vi "LEDS.vi"(7 "Action":T1, 8 "error in":errorcluster, 10 "On/Off":bool) -> (0 "error out":errorcluster)   [LabVIEW 2015]
uses:
  LEDSaction.ctl
  <vilib>/Rock Robotics/SystemInterfaces/DIO/FPGA_DIOChannel.ctl
  <vilib>/Rock Robotics/SystemInterfaces/Typedef/FPGA_TypedefDigitalModule.ctl
panel:
  out "PressureHigh":bool
  out "PressureLow":bool
  out "Shoot":bool
  out "Shift":bool
  out "Hot":bool
  out "NotHot":bool
  out "10 Seconds":bool
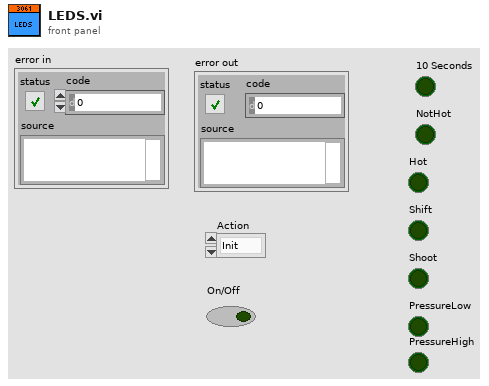
[diagram p1: front panel]
types:
  T1 = typedef "LEDSaction.ctl" = enum16{"Init", "10SecondsLeft", "LimitDown", "LimitUp", "CollectDown", "CollectUp", "NotHot", "Hot", "Shift", "RollBack", "RollFwd", "Shoot", "Distance Low", "DistanceHigh", "PressureLow", "PressureHigh"}
  T2 = typedef "FPGA_DIOChannel.ctl" = enum8{"DIO 1", "DIO 2", "DIO 3", "DIO 4", "DIO 5", "DIO 6", "DIO 7", "DIO 8", "DIO 9", "DIO 10", "DIO 11", "DIO 12", "DIO 13", "DIO 14", "Invalid"}
  T3 = typedef "FPGA_TypedefDigitalModule.ctl" = enum16{"Digital Module 1", "Digital Module 2"}
  T4 = typedef "WPI_DigitalOutputDevRef.ctl" = cluster{"Digital Module":T3, "DIO Channel":T2, "DevStatus":errorcluster}
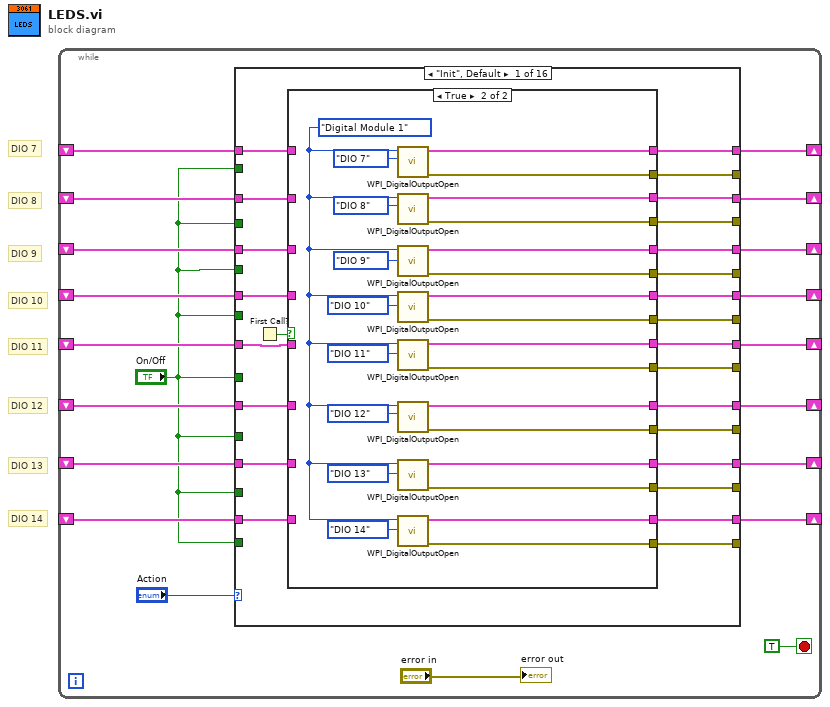
[diagram p0: block diagram]
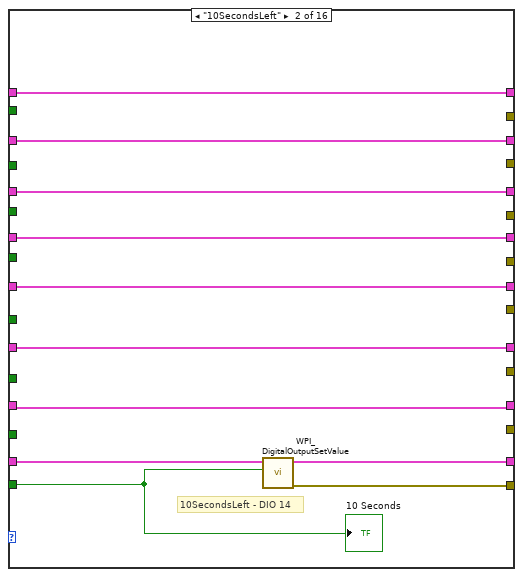
[diagram p3: hidden frame]
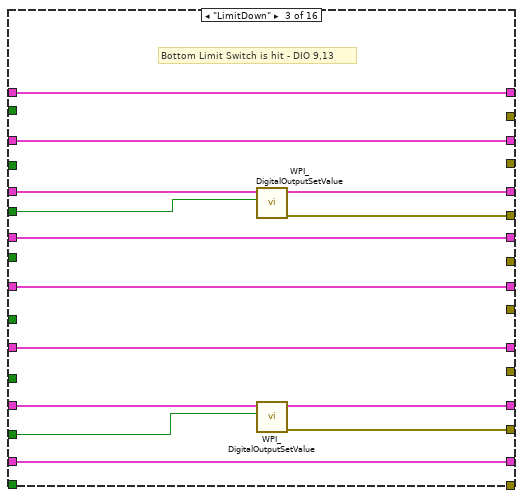
[diagram p4: hidden frame]
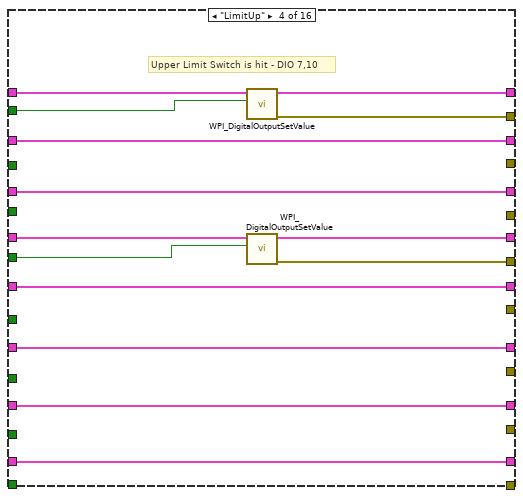
[diagram p5: hidden frame]
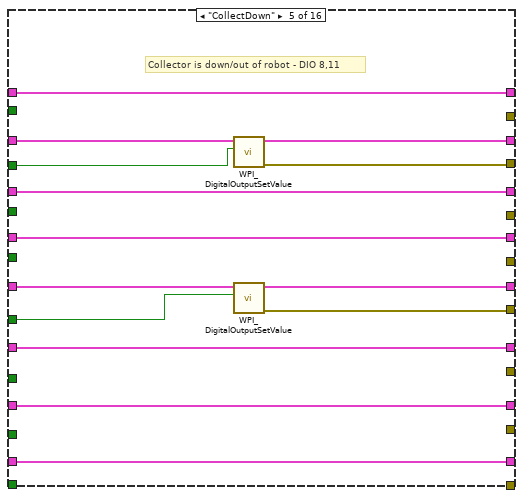
[diagram p6: hidden frame]
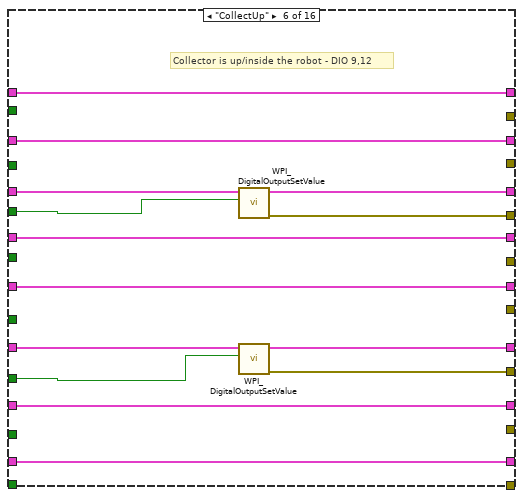
[diagram p7: hidden frame]
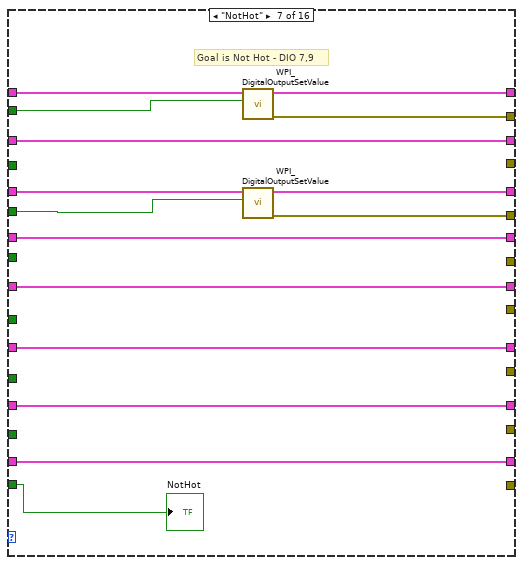
[diagram p8: hidden frame]
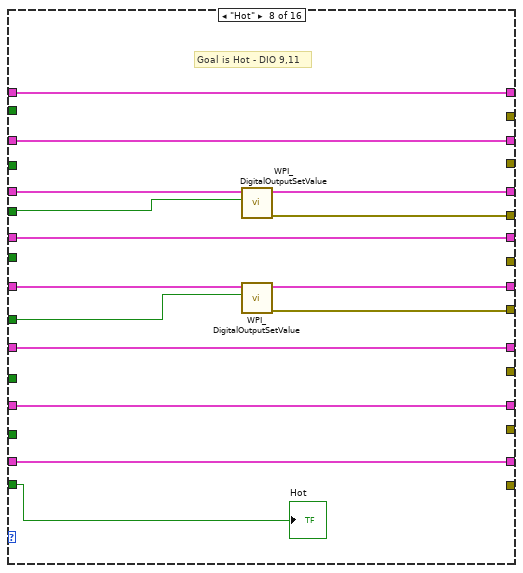
[diagram p9: hidden frame]
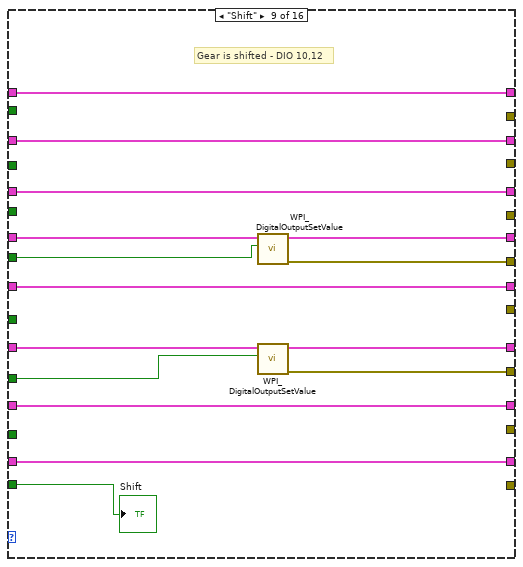
[diagram p10: hidden frame]
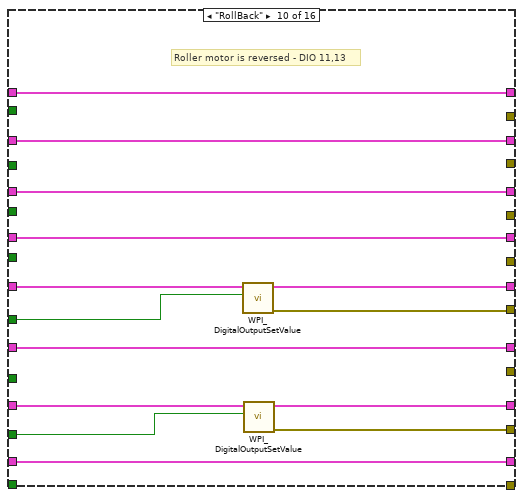
[diagram p11: hidden frame]
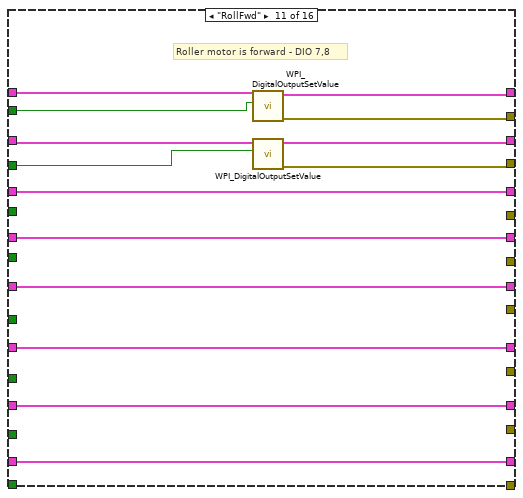
[diagram p12: hidden frame]
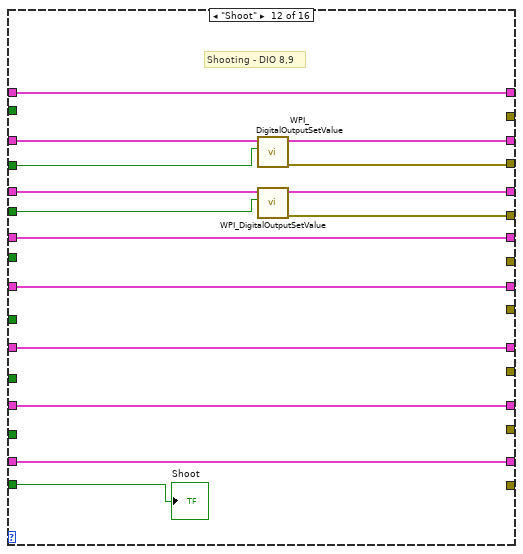
[diagram p13: hidden frame]
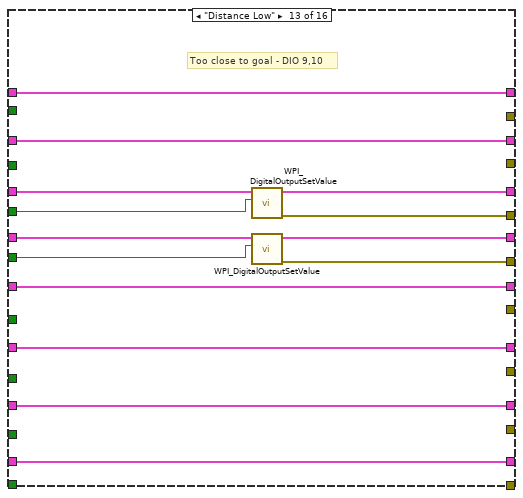
[diagram p14: hidden frame]
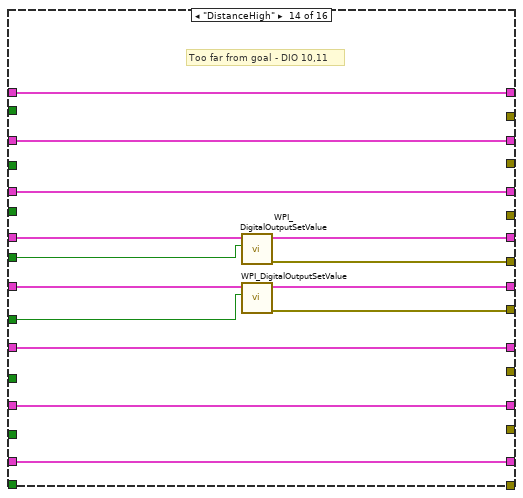
[diagram p15: hidden frame]
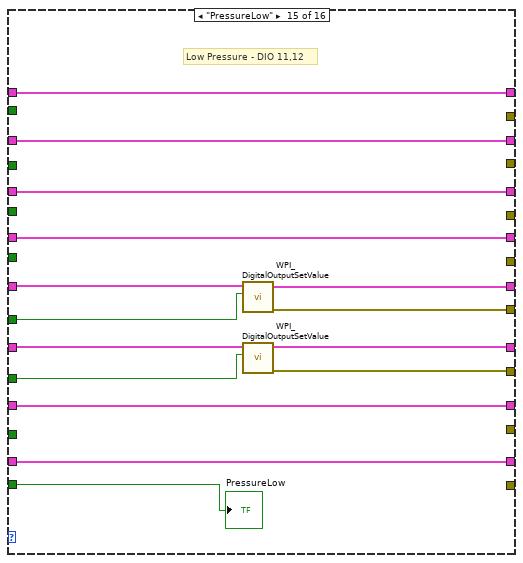
[diagram p16: hidden frame]
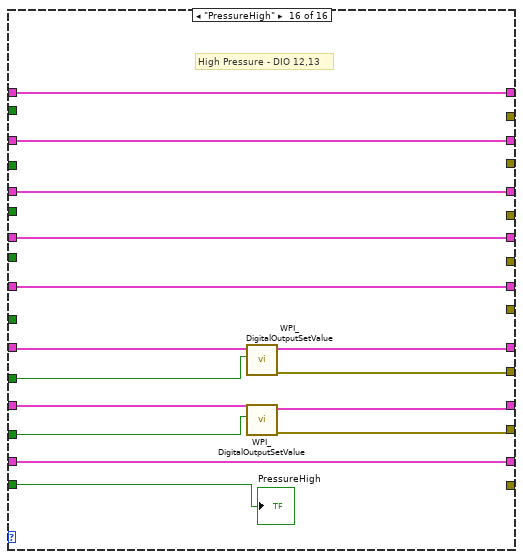
[diagram p17: hidden frame]
diagram:
  # "DIO 14"
  # "DIO 13"
  # "DIO 12"
  # "DIO 11"
  # "DIO 10"
  # "DIO 9"
  # "DIO 8"
  # "DIO 7"
  n1 = while {
    shift-right: [w20] -> _
    shift-left: _ -> [w12]
    shift-right: [w19] -> _
    shift-left: _ -> [w11]
    shift-right: [w18] -> _
    shift-left: _ -> [w10]
    shift-right: [w17] -> _
    shift-left: _ -> [w9]
    shift-right: [w16] -> _
    shift-left: _ -> [w8]
    shift-right: [w15] -> _
    shift-left: _ -> [w7]
    shift-right: [w14] -> _
    shift-left: _ -> [w6]
    shift-right: [w13] -> _
    shift-left: _ -> [w5]
    stop <- TRUE stop-if-true
    n2 = case shown="\"Init\", Default" "Action" {
      tunnel: [w30 w87 w94 w117 w127 w141 w159 w169 w183 w195 w218 w229 w243 w255 w267 w282] -> w20
      tunnel: [w32 w86 w95 w112 w131 w140 w156 w170 w184 w196 w217 w233 w242 w256 w268 w283] -> w19
      tunnel: [w34 w85 w102 w113 w126 w145 w160 w175 w185 w197 w214 w232 w247 w257 w269 w284] -> w18
      tunnel: [w36 w84 w96 w116 w125 w139 w155 w171 w189 w198 w213 w228 w246 w260 w270 w285] -> w17
      tunnel: [w38 w83 w97 w111 w130 w138 w154 w174 w186 w203 w212 w227 w241 w261 w275 w286] -> w16
      tunnel: [w40 w82 w98 w110 w124 w144 w153 w168 w190 w200 w211 w226 w240 w254 w276 w290] -> w15
      tunnel: [w42 w81 w101 w109 w123 w137 w152 w167 w182 w204 w210 w225 w239 w253 w272 w291] -> w14
      tunnel: [w44 w88 w99 w108 w122 w136 w151 w166 w181 w199 w209 w224 w238 w252 w271 w287] -> w13
      tunnel: w12 -> [w21 w87 w94 w115 w127 w141 w158 w169 w183 w195 w215 w229 w243 w255 w267 w282]
      tunnel: w11 -> [w22 w86 w95 w112 w128 w140 w156 w170 w184 w196 w216 w230 w242 w256 w268 w283]
      tunnel: w10 -> [w23 w85 w103 w113 w126 w142 w157 w173 w185 w197 w214 w231 w244 w257 w269 w284]
      tunnel: w9 -> [w24 w84 w96 w114 w125 w139 w155 w171 w188 w198 w213 w228 w245 w259 w270 w285]
      tunnel: w8 -> [w28 w83 w97 w111 w129 w138 w154 w172 w186 w201 w212 w227 w241 w258 w274 w286]
      tunnel: w7 -> [w27 w82 w98 w110 w124 w143 w153 w168 w187 w200 w211 w226 w240 w254 w273 w289]
      tunnel: w6 -> [w26 w81 w100 w109 w123 w137 w152 w167 w182 w202 w210 w225 w239 w253 w272 w288]
      tunnel: w5 -> [w25 w89 w99 w108 w122 w136 w151 w166 w181 w199 w209 w224 w238 w252 w271 w287]
      tunnel: [w31 _ _ w107 _ _ w150 _ _ _ w208 _ _ _ _ _] -> _
      tunnel: [w33 _ _ _ w121 _ _ _ _ _ w207 w223 _ _ _ _] -> _
      tunnel: [w35 _ w93 _ _ w135 w149 w165 _ _ _ w222 w237 _ _ _] -> _
      tunnel: [w37 _ _ w106 _ _ _ _ w180 _ _ _ w236 w251 _ _] -> _
      tunnel: [w39 _ _ _ w120 _ _ w164 _ w194 _ _ _ w250 w266 _] -> _
      tunnel: [w41 _ _ _ _ w134 _ _ w179 _ _ _ _ _ w265 w281] -> _
      tunnel: [w43 _ w92 _ _ _ _ _ _ w193 _ _ _ _ _ w280] -> _
      tunnel: [w45 w80 _ _ _ _ _ _ _ _ _ _ _ _ _ _] -> _
      tunnel: "On/Off" -> [_ _ _ _ w118 _ _ w162 _ w192 _ _ _ w248 w264 _]
      tunnel: "On/Off" -> [_ _ _ w105 _ _ w148 _ _ _ w205 _ _ _ _ _]
      tunnel: "On/Off" -> [_ _ _ _ w119 _ _ _ _ _ w206 w221 _ _ _ _]
      tunnel: "On/Off" -> [_ _ w90 _ _ w133 w147 w163 _ _ _ w220 w235 _ _ _]
      tunnel: "On/Off" -> [_ _ _ w104 _ _ _ _ w178 _ _ _ w234 w249 _ _]
      tunnel: "On/Off" -> [_ w79 _ _ _ _ w146 w161 w176 _ _ w219 _ _ w262 w277]
      tunnel: "On/Off" -> [_ _ w91 _ _ _ _ _ _ w191 _ _ _ _ _ w278]
      tunnel: "On/Off" -> [_ _ _ _ _ w132 _ _ w177 _ _ _ _ _ w263 w279]
      frame "Init", Default {
        n3 = First Call?() -> (First Call?: T/F=w29:bool)
        n4 = case shown="True" w29 {
          tunnel: [_ w70] -> w45
          tunnel: [w50 w69] -> w44
          tunnel: [_ w68] -> w43
          tunnel: [w51 w67] -> w42
          tunnel: [_ w66] -> w41
          tunnel: [w52 w65] -> w40
          tunnel: [_ w64] -> w39
          tunnel: [w53 w63] -> w38
          tunnel: [_ w62] -> w37
          tunnel: [w49 w61] -> w36
          tunnel: [_ w60] -> w35
          tunnel: [w48 w59] -> w34
          tunnel: [_ w58] -> w33
          tunnel: [w47 w57] -> w32
          tunnel: [_ w56] -> w31
          tunnel: [w46 w55] -> w30
          tunnel: w28 -> [w53 _]
          tunnel: w27 -> [w52 _]
          tunnel: w26 -> [w51 _]
          tunnel: w25 -> [w50 _]
          tunnel: w24 -> [w49 _]
          tunnel: w23 -> [w48 _]
          tunnel: w22 -> [w47 _]
          tunnel: w21 -> [w46 _]
          frame False {
          }
          frame True {
            w54 = FPGA_TypedefDigitalModule."Digital Module 1" ("Digital Module (Module 1)")
            n5 = call <vilib>:"WPI_DigitalOutputOpen.vi"("DIO Channel"=FPGA_DIOChannel."DIO 7", "Digital Module (Module 1)"=w54) -> ("error out"=w56:errorcluster, "DigitalOutputDevRef"=w55:T4)  [unwired: 8 in]
            n6 = call <vilib>:"WPI_DigitalOutputOpen.vi"("DIO Channel"=FPGA_DIOChannel."DIO 8", "Digital Module (Module 1)"=w54) -> ("error out"=w58:errorcluster, "DigitalOutputDevRef"=w57:T4)  [unwired: 8 in]
            n7 = call <vilib>:"WPI_DigitalOutputOpen.vi"("DIO Channel"=FPGA_DIOChannel."DIO 9", "Digital Module (Module 1)"=w54) -> ("error out"=w60:errorcluster, "DigitalOutputDevRef"=w59:T4)  [unwired: 8 in]
            n8 = call <vilib>:"WPI_DigitalOutputOpen.vi"("DIO Channel"=FPGA_DIOChannel."DIO 10", "Digital Module (Module 1)"=w54) -> ("error out"=w62:errorcluster, "DigitalOutputDevRef"=w61:T4)  [unwired: 8 in]
            n9 = call <vilib>:"WPI_DigitalOutputOpen.vi"("DIO Channel"=FPGA_DIOChannel."DIO 11", "Digital Module (Module 1)"=w54) -> ("error out"=w64:errorcluster, "DigitalOutputDevRef"=w63:T4)  [unwired: 8 in]
            n10 = call <vilib>:"WPI_DigitalOutputOpen.vi"("DIO Channel"=FPGA_DIOChannel."DIO 12", "Digital Module (Module 1)"=w54) -> ("error out"=w66:errorcluster, "DigitalOutputDevRef"=w65:T4)  [unwired: 8 in]
            n11 = call <vilib>:"WPI_DigitalOutputOpen.vi"("DIO Channel"=FPGA_DIOChannel."DIO 13", "Digital Module (Module 1)"=w54) -> ("error out"=w68:errorcluster, "DigitalOutputDevRef"=w67:T4)  [unwired: 8 in]
            n12 = call <vilib>:"WPI_DigitalOutputOpen.vi"("DIO Channel"=FPGA_DIOChannel."DIO 14", "Digital Module (Module 1)"=w54) -> ("error out"=w70:errorcluster, "DigitalOutputDevRef"=w69:T4)  [unwired: 8 in]
          }
        }
      }
      frame "10SecondsLeft" {
        # "10SecondsLeft - DIO 14"
        n13 = call <vilib>:"WPI_DigitalOutputSetValue.vi"("Value"=w79, "DigitalOutputDevRef"=w89) -> ("error out"=w80:errorcluster, "DigitalOutputDevRef"=w88:T4)  [unwired: 8 in]
        "10 Seconds" <- w79
      }
      frame "LimitDown" {
        # "Bottom Limit Switch is hit - DIO 9,13"
        n14 = call <vilib>:"WPI_DigitalOutputSetValue.vi"("Value"=w90, "DigitalOutputDevRef"=w103) -> ("error out"=w93:errorcluster, "DigitalOutputDevRef"=w102:T4)  [unwired: 8 in]
        n15 = call <vilib>:"WPI_DigitalOutputSetValue.vi"("Value"=w91, "DigitalOutputDevRef"=w100) -> ("error out"=w92:errorcluster, "DigitalOutputDevRef"=w101:T4)  [unwired: 8 in]
      }
      frame "LimitUp" {
        # "Upper Limit Switch is hit - DIO 7,10"
        n16 = call <vilib>:"WPI_DigitalOutputSetValue.vi"("Value"=w105, "DigitalOutputDevRef"=w115) -> ("error out"=w107:errorcluster, "DigitalOutputDevRef"=w117:T4)  [unwired: 8 in]
        n17 = call <vilib>:"WPI_DigitalOutputSetValue.vi"("Value"=w104, "DigitalOutputDevRef"=w114) -> ("error out"=w106:errorcluster, "DigitalOutputDevRef"=w116:T4)  [unwired: 8 in]
      }
      frame "CollectDown" {
        # "Collector is down/out of robot - DIO 8,11"
        n18 = call <vilib>:"WPI_DigitalOutputSetValue.vi"("Value"=w119, "DigitalOutputDevRef"=w128) -> ("error out"=w121:errorcluster, "DigitalOutputDevRef"=w131:T4)  [unwired: 8 in]
        n19 = call <vilib>:"WPI_DigitalOutputSetValue.vi"("Value"=w118, "DigitalOutputDevRef"=w129) -> ("error out"=w120:errorcluster, "DigitalOutputDevRef"=w130:T4)  [unwired: 8 in]
      }
      frame "CollectUp" {
        # "Collector is up/inside the robot - DIO 9,12"
        n20 = call <vilib>:"WPI_DigitalOutputSetValue.vi"("Value"=w133, "DigitalOutputDevRef"=w142) -> ("error out"=w135:errorcluster, "DigitalOutputDevRef"=w145:T4)  [unwired: 8 in]
        n21 = call <vilib>:"WPI_DigitalOutputSetValue.vi"("Value"=w132, "DigitalOutputDevRef"=w143) -> ("error out"=w134:errorcluster, "DigitalOutputDevRef"=w144:T4)  [unwired: 8 in]
      }
      frame "NotHot" {
        # "Goal is Not Hot - DIO 7,9"
        n22 = call <vilib>:"WPI_DigitalOutputSetValue.vi"("Value"=w148, "DigitalOutputDevRef"=w158) -> ("error out"=w150:errorcluster, "DigitalOutputDevRef"=w159:T4)  [unwired: 8 in]
        n23 = call <vilib>:"WPI_DigitalOutputSetValue.vi"("Value"=w147, "DigitalOutputDevRef"=w157) -> ("error out"=w149:errorcluster, "DigitalOutputDevRef"=w160:T4)  [unwired: 8 in]
        "NotHot" <- w146
      }
      frame "Hot" {
        # "Goal is Hot - DIO 9,11"
        n24 = call <vilib>:"WPI_DigitalOutputSetValue.vi"("Value"=w163, "DigitalOutputDevRef"=w173) -> ("error out"=w165:errorcluster, "DigitalOutputDevRef"=w175:T4)  [unwired: 8 in]
        n25 = call <vilib>:"WPI_DigitalOutputSetValue.vi"("Value"=w162, "DigitalOutputDevRef"=w172) -> ("error out"=w164:errorcluster, "DigitalOutputDevRef"=w174:T4)  [unwired: 8 in]
        "Hot" <- w161
      }
      frame "Shift" {
        # "Gear is shifted - DIO 10,12"
        n26 = call <vilib>:"WPI_DigitalOutputSetValue.vi"("Value"=w178, "DigitalOutputDevRef"=w188) -> ("error out"=w180:errorcluster, "DigitalOutputDevRef"=w189:T4)  [unwired: 8 in]
        n27 = call <vilib>:"WPI_DigitalOutputSetValue.vi"("Value"=w177, "DigitalOutputDevRef"=w187) -> ("error out"=w179:errorcluster, "DigitalOutputDevRef"=w190:T4)  [unwired: 8 in]
        "Shift" <- w176
      }
      frame "RollBack" {
        # "Roller motor is reversed - DIO 11,13"
        n28 = call <vilib>:"WPI_DigitalOutputSetValue.vi"("Value"=w192, "DigitalOutputDevRef"=w201) -> ("error out"=w194:errorcluster, "DigitalOutputDevRef"=w203:T4)  [unwired: 8 in]
        n29 = call <vilib>:"WPI_DigitalOutputSetValue.vi"("Value"=w191, "DigitalOutputDevRef"=w202) -> ("error out"=w193:errorcluster, "DigitalOutputDevRef"=w204:T4)  [unwired: 8 in]
      }
      frame "RollFwd" {
        # "Roller motor is forward - DIO 7,8"
        n30 = call <vilib>:"WPI_DigitalOutputSetValue.vi"("Value"=w205, "DigitalOutputDevRef"=w215) -> ("error out"=w208:errorcluster, "DigitalOutputDevRef"=w218:T4)  [unwired: 8 in]
        n31 = call <vilib>:"WPI_DigitalOutputSetValue.vi"("Value"=w206, "DigitalOutputDevRef"=w216) -> ("error out"=w207:errorcluster, "DigitalOutputDevRef"=w217:T4)  [unwired: 8 in]
      }
      frame "Shoot" {
        # "Shooting - DIO 8,9"
        n32 = call <vilib>:"WPI_DigitalOutputSetValue.vi"("Value"=w221, "DigitalOutputDevRef"=w230) -> ("error out"=w223:errorcluster, "DigitalOutputDevRef"=w233:T4)  [unwired: 8 in]
        n33 = call <vilib>:"WPI_DigitalOutputSetValue.vi"("Value"=w220, "DigitalOutputDevRef"=w231) -> ("error out"=w222:errorcluster, "DigitalOutputDevRef"=w232:T4)  [unwired: 8 in]
        "Shoot" <- w219
      }
      frame "Distance Low" {
        # "Too close to goal - DIO 9,10"
        n34 = call <vilib>:"WPI_DigitalOutputSetValue.vi"("Value"=w235, "DigitalOutputDevRef"=w244) -> ("error out"=w237:errorcluster, "DigitalOutputDevRef"=w247:T4)  [unwired: 8 in]
        n35 = call <vilib>:"WPI_DigitalOutputSetValue.vi"("Value"=w234, "DigitalOutputDevRef"=w245) -> ("error out"=w236:errorcluster, "DigitalOutputDevRef"=w246:T4)  [unwired: 8 in]
      }
      frame "DistanceHigh" {
        # "Too far from goal - DIO 10,11"
        n36 = call <vilib>:"WPI_DigitalOutputSetValue.vi"("Value"=w249, "DigitalOutputDevRef"=w259) -> ("error out"=w251:errorcluster, "DigitalOutputDevRef"=w260:T4)  [unwired: 8 in]
        n37 = call <vilib>:"WPI_DigitalOutputSetValue.vi"("Value"=w248, "DigitalOutputDevRef"=w258) -> ("error out"=w250:errorcluster, "DigitalOutputDevRef"=w261:T4)  [unwired: 8 in]
      }
      frame "PressureLow" {
        # "Low Pressure - DIO 11,12"
        n38 = call <vilib>:"WPI_DigitalOutputSetValue.vi"("Value"=w264, "DigitalOutputDevRef"=w274) -> ("error out"=w266:errorcluster, "DigitalOutputDevRef"=w275:T4)  [unwired: 8 in]
        n39 = call <vilib>:"WPI_DigitalOutputSetValue.vi"("Value"=w263, "DigitalOutputDevRef"=w273) -> ("error out"=w265:errorcluster, "DigitalOutputDevRef"=w276:T4)  [unwired: 8 in]
        "PressureLow" <- w262
      }
      frame "PressureHigh" {
        # "High Pressure - DIO 12,13"
        n40 = call <vilib>:"WPI_DigitalOutputSetValue.vi"("Value"=w279, "DigitalOutputDevRef"=w289) -> ("error out"=w281:errorcluster, "DigitalOutputDevRef"=w290:T4)  [unwired: 8 in]
        n41 = call <vilib>:"WPI_DigitalOutputSetValue.vi"("Value"=w278, "DigitalOutputDevRef"=w288) -> ("error out"=w280:errorcluster, "DigitalOutputDevRef"=w291:T4)  [unwired: 8 in]
        "PressureHigh" <- w277
      }
    }
    "error out" <- "error in"
  }
